vi "Close.vi"(8 "error in (no error)":errorcluster, 11 "User Connections in":refnum<class "User Connections.lvclass">) -> (0 "error out":errorcluster)   [LabVIEW 2025, in "File Library.lvlib" / "User Connections.lvclass"]
uses:
  User Connections.lvclass
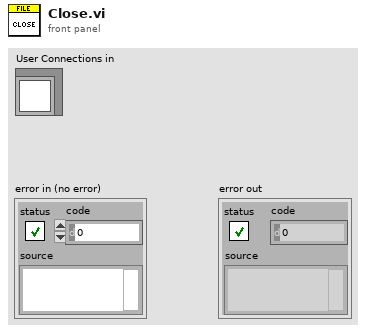
[diagram p1: front panel]
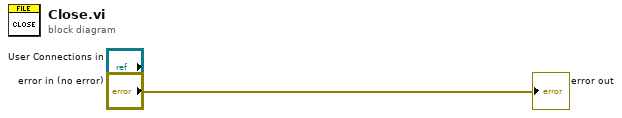
[diagram p0: block diagram]
diagram:
  "error out" <- "error in (no error)"
